vi "抓邊.vi"() -> ()   [LabVIEW 2015]
uses:
  <vilib>/vision/Measure.llb/Edge Options.ctl
  <vilib>/vision/Measure.llb/Edge Polarity.ctl
  <vilib>/vision/NI_Vision_Development_Module.lvlib
panel:
  out "degrees":sgl
  in  "單點":bool
  in  "Edge Options":T1={"Edge Polarity"=0, "Kernel Size"=3, "Width"=3, "Minimum Edge Strength"=10.0, "Interpolation Type"=enum."Bilinear Fixed", "Data Processing Method"=enum."Average"} {"Edge Polarity" items=["All Edges", "Rising Edges", "Falling Edges"]; "Minimum Edge Strength" format="%.2f"; "Width" step=2; "Kernel Size" step=2}
  in  "開圖":bool
  out "Gradient Information":dbl[][](graph)
  out "Line Segment":T3 {"Point 2"."Y" format="%.2f"; "Point 2"."X" format="%.2f"; "Point 1"."Y" format="%.2f"; "Point 1"."X" format="%.2f"}
  out "error out":errorcluster
  in  "Direction":T4(ring)
  in  "Process":u16(ring) items=["Get First Edge", "Get First + Last Edge", "Get All Edges", "Get Best Edge"]
  out "Line Profile":T5(graph)
  in  "Gap":i32=10
  out "Image":T6(plugin-control)
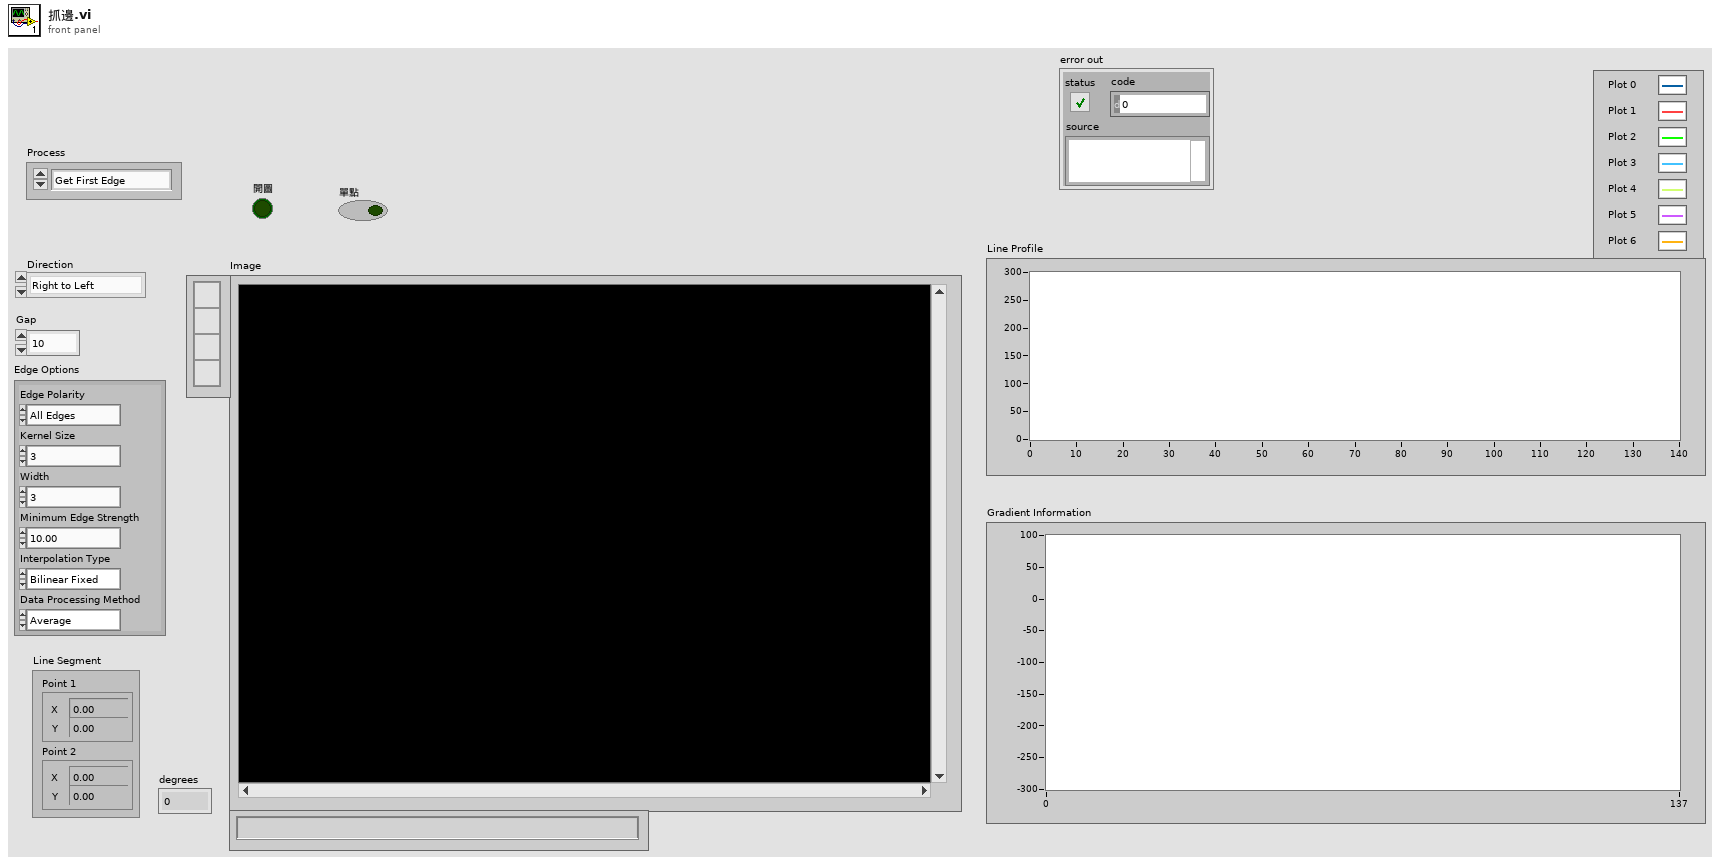
[diagram p1: front panel]
types:
  T1 = typedef "Edge Options.ctl" = cluster{"Edge Polarity":T2, "Kernel Size":u32, "Width":u32, "Minimum Edge Strength":sgl, "Interpolation Type":enum32{"Zero Order", "Bilinear", "Quadratic", "Cubic", "Bilinear Fixed"}, "Data Processing Method":enum32{"Average", "Median"}}
  T2 = typedef "Edge Polarity.ctl" = u32
  T3 = cluster{"Point 1":cluster{"X":sgl, "Y":sgl}, "Point 2":cluster{"X":sgl, "Y":sgl}}
  T4 = enum16{"Right to Left", "Left  to Right", "Up to Down", "Down to Up"}
  T5 = cluster{"x0":sgl, "dx":sgl, "Pixels Line":sgl[]}[]
  T6 = typedef "IMAQ Image.ctl" = refnum<image>
  T7 = typedef "Image Type" = u32
  T8 = cluster{"Global Rectangle":i32[], "Contours":cluster{"Contour Type":u32, "ROI Type":u32, "Points":i32[]}[]}
  T9 = typedef "IMAQ Line" = cluster{"Start X":i32, "Start Y":i32, "End X":i32, "End Y":i32}
  T10 = typedef "IMAQ Rectangle" = cluster{"Left":i32, "Top":i32, "Right":i32, "Bottom":i32, "Rotation":dbl}
  T11 = typedef "IMAQ Point" = cluster{"X":sgl, "Y":sgl}
  T12 = typedef "ROI Descriptor" = cluster{"Global Rectangle":i32[], "Contours":cluster{"ID":enum32{"External", "Internal"}, "Type":u32, "Coordinates":i32[]}[]}
  T13 = typedef "Edge New.ctl" = cluster{"Location (Pixel)":cluster{"X":sgl, "Y":sgl}, "Location (Real-World)":cluster{"X":sgl, "Y":sgl}, "Distance (Pixel)":dbl, "Distance (Real-World)":dbl, "Strength":dbl, "Noise":dbl, "Rising?":bool}
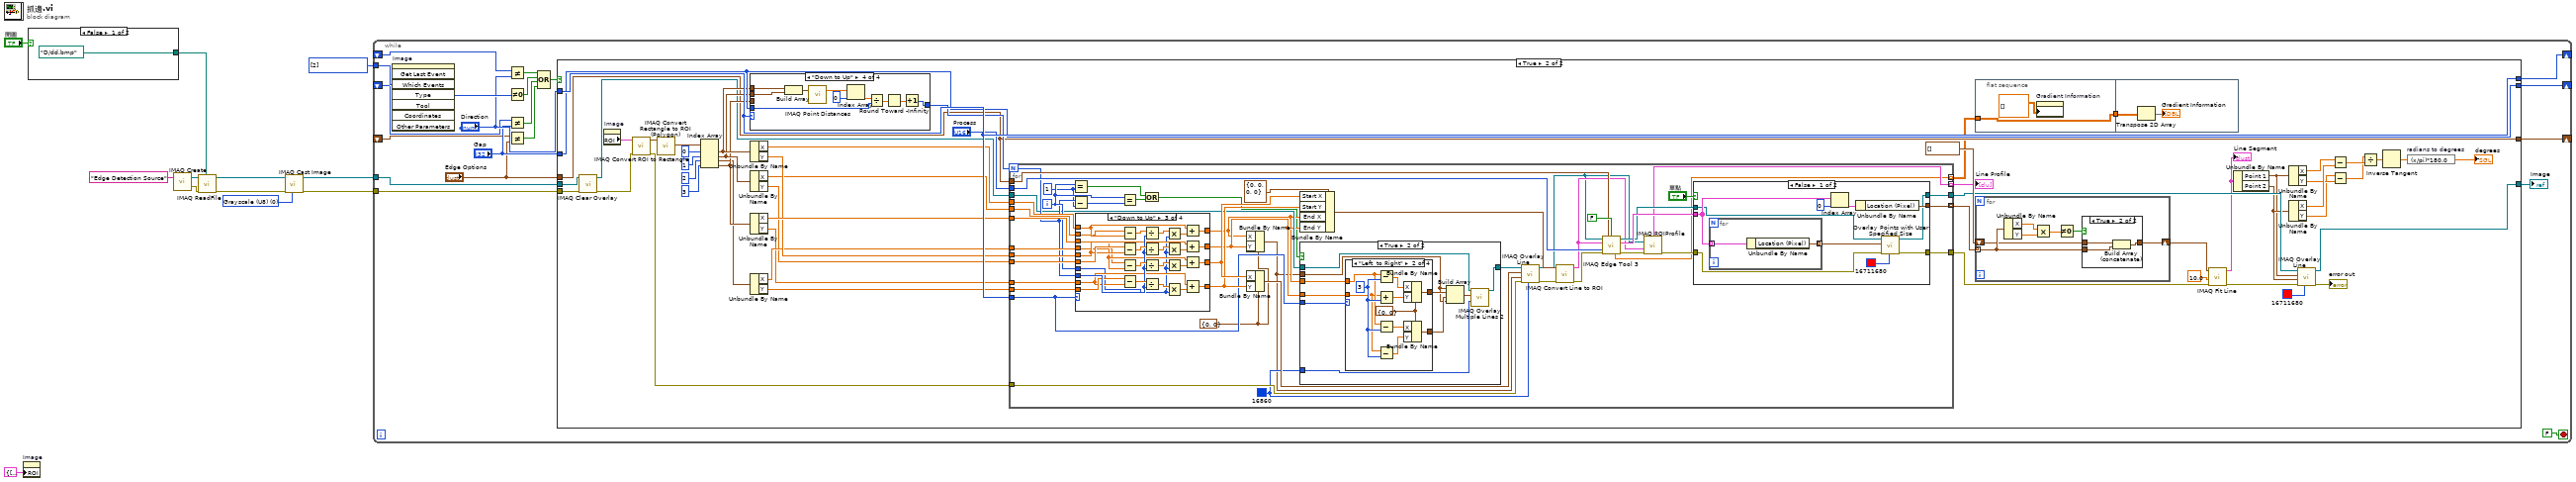
[diagram p0: block diagram]
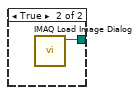
[diagram p2: hidden frame]
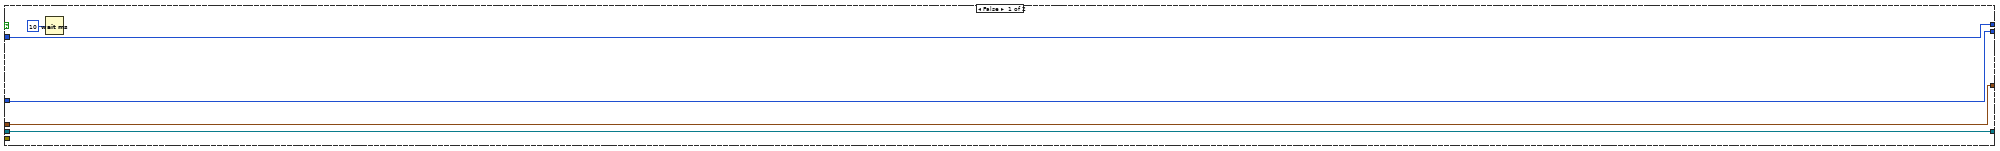
[diagram p3: hidden frame]
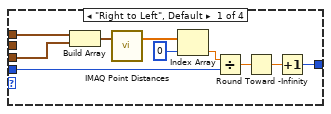
[diagram p4: hidden frame]
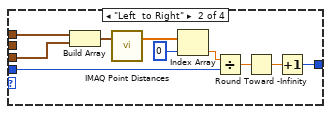
[diagram p5: hidden frame]
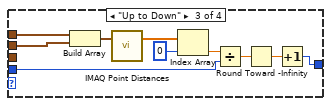
[diagram p6: hidden frame]
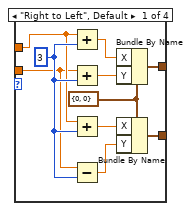
[diagram p9: hidden frame]
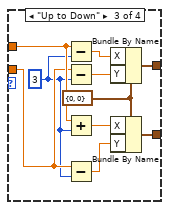
[diagram p10: hidden frame]
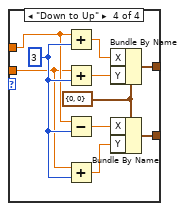
[diagram p11: hidden frame]
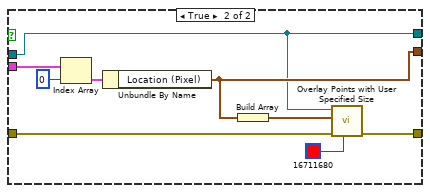
[diagram p12: hidden frame]
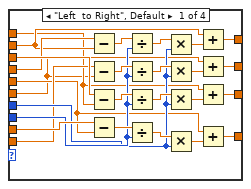
[diagram p13: hidden frame]
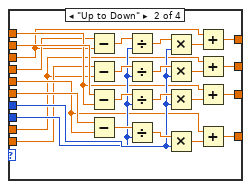
[diagram p14: hidden frame]
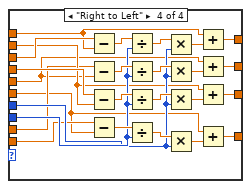
[diagram p15: hidden frame]
diagram:
  w6 = T7 0 items=["Grayscale (U8)", "Grayscale (I16)", "Grayscale (SGL)", "Complex (CSG)", "RGB (U32)", "HSL (U32)", "RGB (U64)", "Grayscale (U16)"] ("Image Type")
  w8 = i32[] [2] items=["No  event", "Click event", "Draw event", "Move event", "Size event", "Scroll event", "Activate event", "Close event", "Double click event"] ("Events list (all)")
  n1 = property on="Image" class="ImageControl"("ROI"=T8 {"Global Rectangle"=[450, 180, 600, 400], "Contours"=[{"Contour Type"=0, "ROI Type"=3, "Points"=[450, 180, 600, 400]}]}) -> ()  [unwired: 2 in, 2 out]
  n2 = case shown="False" "開圖" {
    tunnel: [path "D:/dd.bmp" ("File Path") w14] -> w3
    frame False {
    }
    frame True {
      n3 = call "IMAQ Load Image Dialog"() -> ("Path"=w14:path)  [unwired: 9 in, 2 out]
    }
  }
  n4 = call "IMAQ Create"("Image Name"="Edge Detection Source") -> ("New Image"=w11:T6, "error out"=w10:errorcluster)  [unwired: 4 in]
  n5 = call "IMAQ ReadFile"("File Path"=w3, "error in (no error)"=w10, "Image"=w11) -> ("error out"=w2:errorcluster, "Image Out"=w5:T6)  [unwired: 4 in, 3 out]
  n6 = call "IMAQ Cast Image"("Image Type"=w6, "error in (no error)"=w2, "Image Src"=w5) -> ("error out"=w1:errorcluster, "Image Dst Out"=w7:T6)  [unwired: 7 in]
  n7 = while {
    tunnel: w1 -> [w32]
    tunnel: w7 -> [w33]
    tunnel: w8 -> [w31]
    shift-right: [w29] -> _
    shift-left: _ -> [w28]
    shift-right: [w21] -> _
    shift-left: _ -> [w22]
    shift-right: [w16] -> _
    shift-left: _ -> [w17]
    stop <- FALSE stop-if-true
    n8 = invoke on="Image" class="ImageControl" method="Get Last Event"("Which Events"=w31) -> ("Type"=w30:i32)  [unwired: 7 in, 7 out]
    n9 = Not Equal?(x=w28, y="Direction") -> (x != y?=w27:bool)
    n10 = Not Equal To 0?(x=w30) -> (x != 0?=w26:bool)
    n11 = Not Equal?(x=w22, y="Gap") -> (x != y?=w20:bool)
    n12 = Not Equal?(x=w17, y="Edge Options") -> (x != y?=w15:bool)
    n13 = Compound Arithmetic op=OR(w27, w26, w20, w15) -> (w25:bool)
    n14 = case shown="True" w25 {
      tunnel: w33 -> [w36 w92]
      tunnel: w32 -> [_ w91]
      tunnel: "Direction" -> [w38 w82]
      tunnel: [w38 w82] -> w29
      tunnel: "Gap" -> [w37 w81]
      tunnel: [w37 w81] -> w21
      tunnel: [w36 w52] -> w19
      tunnel: "Edge Options" -> [w35 w61]
      tunnel: [w35 w61] -> w16
      frame False {
        n15 = Wait (ms)(milliseconds to wait=u32 10) -> ()  [unwired: 1 out]
      }
      frame True {
        n16 = call "IMAQ Clear Overlay"("error in (no error)"=w91, "Image"=w92) -> ("error out"=w90:errorcluster, "Image Out"=w64:T6)  [unwired: 8 in]
        n17 = property on="Image" class="ImageControl"() -> ("ROI"=w93:T8)  [unwired: 2 in, 2 out]
        n18 = call "IMAQ Convert ROI to Rectangle"("error in (no error)"=w90, "ROI Descriptor"=w93) -> ("error out"=w63:errorcluster, "Rectangle"=w85:T10)  [unwired: 7 in]
        n19 = call "IMAQ Convert Rectangle to ROI (Polygon)"("Rectangle"=w85) -> ("Rectangle Points"=w78:T11[])  [unwired: 7 in, 2 out]
        n20 = Index Array(array=w78, index #1=0 ("index"), index #2=1 ("index"), index #3=2 ("index"), index #4=3 ("index")) -> (element #1=w80:T11, element #2=w79:T11, element #3=w70:T11, element #4=w71:T11)
        n21 = case shown="\"Down to Up\"" w82 {
          tunnel: w81 -> [w101 w111 w121 w131]
          tunnel: [w100 w110 w120 w130] -> w77
          tunnel: w80 -> [w97 w107 w119 w127]
          tunnel: w71 -> [w96 w106 _ _]
          tunnel: w79 -> [_ _ w115 w126]
          frame "Right to Left", Default {
            n22 = Build Array(w97, w96) -> (w99:T11[])
            n23 = call "IMAQ Point Distances"("Points"=w99) -> ("Distances"=w98:sgl[])  [unwired: 4 in, 1 out]
            n24 = Index Array(array=w98, index=0) -> (element=w94:sgl)
            n25 = Divide(x=w94, y=w101) -> (x/y=w102:sgl)
            n26 = Round Toward -Infinity(1:w102) -> (0:w103:sgl)
            n27 = Increment(x=w103) -> (x+1=w100:i32)
          }
          frame "Left  to Right" {
            n28 = Build Array(w107, w106) -> (w109:T11[])
            n29 = call "IMAQ Point Distances"("Points"=w109) -> ("Distances"=w108:sgl[])  [unwired: 4 in, 1 out]
            n30 = Index Array(array=w108, index=0) -> (element=w104:sgl)
            n31 = Divide(x=w104, y=w111) -> (x/y=w112:sgl)
            n32 = Round Toward -Infinity(1:w112) -> (0:w113:sgl)
            n33 = Increment(x=w113) -> (x+1=w110:i32)
          }
          frame "Up to Down" {
            n34 = Build Array(w119, w115) -> (w118:T11[])
            n35 = call "IMAQ Point Distances"("Points"=w118) -> ("Distances"=w117:sgl[])  [unwired: 4 in, 1 out]
            n36 = Index Array(array=w117, index=0) -> (element=w116:sgl)
            n37 = Divide(x=w116, y=w121) -> (x/y=w122:sgl)
            n38 = Round Toward -Infinity(1:w122) -> (0:w123:sgl)
            n39 = Increment(x=w123) -> (x+1=w120:i32)
          }
          frame "Down to Up" {
            n40 = Build Array(w127, w126) -> (w129:T11[])
            n41 = call "IMAQ Point Distances"("Points"=w129) -> ("Distances"=w128:sgl[])  [unwired: 4 in, 1 out]
            n42 = Index Array(array=w128, index=0) -> (element=w125:sgl)
            n43 = Divide(x=w125, y=w131) -> (x/y=w132:sgl)
            n44 = Round Toward -Infinity(1:w132) -> (0:w133:sgl)
            n45 = Increment(x=w133) -> (x+1=w130:i32)
          }
        }
        n46 = Unbundle By Name(w80) -> ("X"=w75:sgl, "Y"=w74:sgl)
        n47 = Unbundle By Name(w79) -> ("X"=w68:sgl, "Y"=w66:sgl)
        n48 = Unbundle By Name(w71) -> ("X"=w76:sgl, "Y"=w65:sgl)
        n49 = Unbundle By Name(w70) -> ("X"=w69:sgl, "Y"=w67:sgl)
        n50 = for {
          N: w77 -> [w163]
          tunnel: w82 -> [w154]
          tunnel: w76 -> [w193]
          tunnel: w75 -> [w192]
          tunnel: w65 -> [w191]
          tunnel: w74 -> [w190]
          tunnel: w69 -> [w189]
          tunnel: w68 -> [w188]
          tunnel: w67 -> [w187]
          tunnel: w66 -> [w186]
          tunnel: [w175] -> w57
          tunnel: w64 -> [w158]
          tunnel: w63 -> [w184]
          tunnel: [w173] -> w56
          tunnel: "Process" -> [w176]
          tunnel: w61 -> [w172]
          tunnel: [w170] -> w60 mode=indexing
          tunnel: [w169] -> w59 mode=indexing
          tunnel: [w168] -> w58 mode=indexing
          i -> [w164]
          w162 = 1
          w156 = u32 16860 ("Color")
          w152 = cluster{"X":i32, "Y":i32} {"X"=0, "Y"=0} ("Start Point")
          n51 = Equal?(x=w164, y=w162) -> (x = y?=w160:bool)
          n52 = Subtract(x=w163, y=w162) -> (x-y=w161:i32)
          n53 = case shown="\"Down to Up\"" w154 {
            tunnel: [w277 w296 w322 w347] -> w183
            tunnel: [w272 w295 w321 w348] -> w151
            tunnel: [w275 w293 w319 w345] -> w182
            tunnel: [w271 w294 w320 w346] -> w153
            tunnel: w193 -> [w290 w301 w327 w357]
            tunnel: w192 -> [w268 w303 w326 w356]
            tunnel: w163 -> [w281 w305 w332 w358]
            tunnel: w164 -> [w280 w306 w323 w355]
            tunnel: w191 -> [w287 w297 w329 w352]
            tunnel: w190 -> [w270 w299 w328 w351]
            tunnel: w189 -> [w284 w302 w325 w354]
            tunnel: w188 -> [w269 w304 w324 w353]
            tunnel: w187 -> [w279 w298 w330 w350]
            tunnel: w186 -> [w267 w300 w331 w349]
            frame "Left  to Right", Default {
              n54 = Subtract(x=w284, y=w269) -> (x-y=w286:sgl)
              n55 = Subtract(x=w279, y=w267) -> (x-y=w282:sgl)
              n56 = Subtract(x=w290, y=w268) -> (x-y=w291:sgl)
              n57 = Subtract(x=w287, y=w270) -> (x-y=w289:sgl)
              n58 = Divide(x=w286, y=w281) -> (x/y=w285:sgl)
              n59 = Divide(x=w282, y=w281) -> (x/y=w283:sgl)
              n60 = Divide(x=w291, y=w281) -> (x/y=w292:sgl)
              n61 = Divide(x=w289, y=w281) -> (x/y=w288:sgl)
              n62 = Multiply(x=w285, y=w280) -> (x*y=w274:sgl)
              n63 = Multiply(x=w283, y=w280) -> (x*y=w273:sgl)
              n64 = Multiply(x=w292, y=w280) -> (x*y=w278:sgl)
              n65 = Multiply(x=w288, y=w280) -> (x*y=w276:sgl)
              n66 = Add(x=w269, y=w274) -> (x+y=w272:sgl)
              n67 = Add(x=w267, y=w273) -> (x+y=w271:sgl)
              n68 = Add(x=w268, y=w278) -> (x+y=w277:sgl)
              n69 = Add(x=w270, y=w276) -> (x+y=w275:sgl)
            }
            frame "Up to Down" {
              n70 = Subtract(x=w302, y=w301) -> (x-y=w314:sgl)
              n71 = Subtract(x=w298, y=w297) -> (x-y=w311:sgl)
              n72 = Subtract(x=w304, y=w303) -> (x-y=w317:sgl)
              n73 = Subtract(x=w300, y=w299) -> (x-y=w316:sgl)
              n74 = Divide(x=w314, y=w305) -> (x/y=w313:sgl)
              n75 = Divide(x=w311, y=w305) -> (x/y=w312:sgl)
              n76 = Divide(x=w317, y=w305) -> (x/y=w318:sgl)
              n77 = Divide(x=w316, y=w305) -> (x/y=w315:sgl)
              n78 = Multiply(x=w313, y=w306) -> (x*y=w308:sgl)
              n79 = Multiply(x=w312, y=w306) -> (x*y=w307:sgl)
              n80 = Multiply(x=w318, y=w306) -> (x*y=w310:sgl)
              n81 = Multiply(x=w315, y=w306) -> (x*y=w309:sgl)
              n82 = Add(x=w301, y=w308) -> (x+y=w295:sgl)
              n83 = Add(x=w297, y=w307) -> (x+y=w294:sgl)
              n84 = Add(x=w303, y=w310) -> (x+y=w296:sgl)
              n85 = Add(x=w299, y=w309) -> (x+y=w293:sgl)
            }
            frame "Down to Up" {
              n86 = Subtract(x=w324, y=w326) -> (x-y=w343:sgl)
              n87 = Subtract(x=w331, y=w328) -> (x-y=w342:sgl)
              n88 = Subtract(x=w325, y=w327) -> (x-y=w340:sgl)
              n89 = Subtract(x=w330, y=w329) -> (x-y=w337:sgl)
              n90 = Divide(x=w343, y=w332) -> (x/y=w344:sgl)
              n91 = Divide(x=w342, y=w332) -> (x/y=w341:sgl)
              n92 = Divide(x=w340, y=w332) -> (x/y=w339:sgl)
              n93 = Divide(x=w337, y=w332) -> (x/y=w338:sgl)
              n94 = Multiply(x=w344, y=w323) -> (x*y=w336:sgl)
              n95 = Multiply(x=w341, y=w323) -> (x*y=w335:sgl)
              n96 = Multiply(x=w339, y=w323) -> (x*y=w334:sgl)
              n97 = Multiply(x=w338, y=w323) -> (x*y=w333:sgl)
              n98 = Add(x=w326, y=w336) -> (x+y=w321:sgl)
              n99 = Add(x=w328, y=w335) -> (x+y=w320:sgl)
              n100 = Add(x=w327, y=w334) -> (x+y=w322:sgl)
              n101 = Add(x=w329, y=w333) -> (x+y=w319:sgl)
            }
            frame "Right to Left" {
              n102 = Subtract(x=w357, y=w356) -> (x-y=w369:sgl)
              n103 = Subtract(x=w352, y=w351) -> (x-y=w368:sgl)
              n104 = Subtract(x=w354, y=w353) -> (x-y=w366:sgl)
              n105 = Subtract(x=w350, y=w349) -> (x-y=w363:sgl)
              n106 = Divide(x=w369, y=w358) -> (x/y=w370:sgl)
              n107 = Divide(x=w368, y=w358) -> (x/y=w367:sgl)
              n108 = Divide(x=w366, y=w358) -> (x/y=w365:sgl)
              n109 = Divide(x=w363, y=w358) -> (x/y=w364:sgl)
              n110 = Multiply(x=w370, y=w355) -> (x*y=w362:sgl)
              n111 = Multiply(x=w367, y=w355) -> (x*y=w361:sgl)
              n112 = Multiply(x=w365, y=w355) -> (x*y=w360:sgl)
              n113 = Multiply(x=w364, y=w355) -> (x*y=w359:sgl)
              n114 = Add(x=w356, y=w362) -> (x+y=w348:sgl)
              n115 = Add(x=w351, y=w361) -> (x+y=w346:sgl)
              n116 = Add(x=w353, y=w360) -> (x+y=w347:sgl)
              n117 = Add(x=w349, y=w359) -> (x+y=w345:sgl)
            }
          }
          n118 = Equal?(x=w164, y=w161) -> (x = y?=w159:bool)
          n119 = Or(x=w160, y=w159) -> (x .or. y?=w149:bool)
          n120 = Bundle By Name(cluster=w152, "X"=w151, "Y"=w153) -> (w150:cluster{"X":i32, "Y":i32})
          n121 = Bundle By Name(cluster=w152, "X"=w183, "Y"=w182) -> (w185:cluster{"X":i32, "Y":i32})
          n122 = Bundle By Name(cluster=T9 {"Start X"=0, "Start Y"=0, "End X"=0, "End Y"=0} ("Line"), "Start X"=w183, "Start Y"=w182, "End X"=w151, "End Y"=w153) -> (w171:T9)
          n123 = case shown="True" w149 {
            tunnel: w158 -> [w195 w205]
            tunnel: [w195 w204] -> w157
            tunnel: w156 -> [_ w203]
            tunnel: w154 -> [_ w202]
            tunnel: w151 -> [_ w196]
            tunnel: w153 -> [_ w201]
            tunnel: w150 -> [_ w197]
            frame False {
            }
            frame True {
              n124 = case shown="\"Left  to Right\"" w202 {
                tunnel: w196 -> [w207 w219 w231 w239]
                tunnel: w201 -> [w206 w218 w230 w238]
                tunnel: [w209 w217 w228 w237] -> w200
                tunnel: [w208 w216 w227 w236] -> w199
                frame "Right to Left", Default {
                  w211 = cluster{"X":i32, "Y":i32} {"X"=0, "Y"=0} ("Start Point")
                  w210 = 3
                  n125 = Add(x=w207, y=w210) -> (x+y=w212:sgl)
                  n126 = Add(x=w206, y=w210) -> (x+y=w213:sgl)
                  n127 = Add(x=w207, y=w210) -> (x+y=w214:sgl)
                  n128 = Subtract(x=w206, y=w210) -> (x-y=w215:sgl)
                  n129 = Bundle By Name(cluster=w211, "X"=w212, "Y"=w213) -> (w209:cluster{"X":i32, "Y":i32})
                  n130 = Bundle By Name(cluster=w211, "X"=w214, "Y"=w215) -> (w208:cluster{"X":i32, "Y":i32})
                }
                frame "Left  to Right" {
                  w221 = cluster{"X":i32, "Y":i32} {"X"=0, "Y"=0} ("Start Point")
                  w220 = 3
                  n131 = Subtract(x=w219, y=w220) -> (x-y=w222:sgl)
                  n132 = Add(x=w218, y=w220) -> (x+y=w223:sgl)
                  n133 = Subtract(x=w219, y=w220) -> (x-y=w224:sgl)
                  n134 = Subtract(x=w218, y=w220) -> (x-y=w225:sgl)
                  n135 = Bundle By Name(cluster=w221, "X"=w222, "Y"=w223) -> (w217:cluster{"X":i32, "Y":i32})
                  n136 = Bundle By Name(cluster=w221, "X"=w224, "Y"=w225) -> (w216:cluster{"X":i32, "Y":i32})
                }
                frame "Up to Down" {
                  w229 = cluster{"X":i32, "Y":i32} {"X"=0, "Y"=0} ("Start Point")
                  w226 = 3
                  n137 = Subtract(x=w231, y=w226) -> (x-y=w232:sgl)
                  n138 = Subtract(x=w230, y=w226) -> (x-y=w233:sgl)
                  n139 = Add(x=w231, y=w226) -> (x+y=w234:sgl)
                  n140 = Subtract(x=w230, y=w226) -> (x-y=w235:sgl)
                  n141 = Bundle By Name(cluster=w229, "X"=w232, "Y"=w233) -> (w228:cluster{"X":i32, "Y":i32})
                  n142 = Bundle By Name(cluster=w229, "X"=w234, "Y"=w235) -> (w227:cluster{"X":i32, "Y":i32})
                }
                frame "Down to Up" {
                  w241 = cluster{"X":i32, "Y":i32} {"X"=0, "Y"=0} ("Start Point")
                  w240 = 3
                  n143 = Add(x=w239, y=w240) -> (x+y=w242:sgl)
                  n144 = Add(x=w238, y=w240) -> (x+y=w243:sgl)
                  n145 = Subtract(x=w239, y=w240) -> (x-y=w244:sgl)
                  n146 = Add(x=w238, y=w240) -> (x+y=w245:sgl)
                  n147 = Bundle By Name(cluster=w241, "X"=w242, "Y"=w243) -> (w237:cluster{"X":i32, "Y":i32})
                  n148 = Bundle By Name(cluster=w241, "X"=w244, "Y"=w245) -> (w236:cluster{"X":i32, "Y":i32})
                }
              }
              n149 = Build Array(w197, w200, w199, w197) -> (w198:cluster{"X":i32, "Y":i32}[])
              n150 = call "IMAQ Overlay Multiple Lines 2"("Image"=w205, "Line End Points"=w198, "Color"=w203) -> ("Image Out"=w204:T6)  [unwired: 11 in, 1 out]
            }
          }
          n151 = call "IMAQ Overlay Line"("Color"=w156, "error in (no error)"=w184, "End Point"=w150, "Start Point"=w185, "Image"=w157) -> ("error out"=w174:errorcluster, "Image Out"=w155:T6)  [unwired: 5 in]
          n152 = call "IMAQ Convert Line to ROI"("error in (no error)"=w174, "Line"=w171) -> ("error out"=w166:errorcluster, "ROI Descriptor"=w165:T12)  [unwired: 7 in]
          n153 = call "IMAQ Edge Tool 3"("Image"=w155, "Edge Options"=w172, "Optimized Mode"=FALSE, "ROI Descriptor"=w165, "Process"=w176, "error in (no error)"=w166) -> ("Image (duplicate)"=w178:T6, "Edge Information"=w181:T13[], "Gradient Values"=w169:dbl[], "error out"=w167:errorcluster)  [unwired: 5 in, 1 out]
          n154 = call "IMAQ ROIProfile"("error in (no error)"=w167, "ROI Descriptor"=w165, "Image"=w155) -> ("error out"=w180:errorcluster, "ROI Graph"=w170:cluster{"x0":sgl, "dx":sgl, "Pixels Line":sgl[]})  [unwired: 1 in, 3 out]
          n155 = case shown="False" "單點" {
            tunnel: [w247 w258] -> w175
            tunnel: w181 -> [w249 w265]
            tunnel: [w252 w262] -> w168
            tunnel: w180 -> [w251 w260]
            tunnel: [w250 w259] -> w173
            tunnel: w178 -> [w246 w258]
            frame False {
              n156 = for {
                tunnel: w249 -> [w257] mode=indexing
                tunnel: [w256] -> w248 mode=indexing
                n157 = Unbundle By Name(w257) -> ("Location (Pixel)"=w256:cluster{"X":sgl, "Y":sgl})
              }
              n158 = Index Array(array=w249, index=0) -> (element=w253:T13)
              n159 = Unbundle By Name(w253) -> ("Location (Pixel)"=w252:cluster{"X":sgl, "Y":sgl})
              n160 = call "Overlay Points with User Specified Size.vi"("Color"=u32 16711680, "error in"=w251, "Points"=w248, "Image In"=w246) -> ("error out"=w250:errorcluster, "Image Out"=w247:T6)  [unwired: 6 in]
            }
            frame True {
              n161 = Index Array(array=w265, index=0) -> (element=w263:T13)
              n162 = Unbundle By Name(w263) -> ("Location (Pixel)"=w262:cluster{"X":sgl, "Y":sgl})
              n163 = Build Array(w262) -> (w261:cluster{"X":sgl, "Y":sgl}[])
              n164 = call "Overlay Points with User Specified Size.vi"("Color"=u32 16711680, "error in"=w260, "Points"=w261, "Image In"=w258) -> ("error out"=w259:errorcluster)  [unwired: 6 in, 1 out]
            }
          }
        }
        "Line Profile" <- w60
        n165 = flat-sequence {
          tunnel: w59 -> [w134]
          tunnel: [w134] -> w86
          tunnel: w86 -> [w136]
          frame #0 {
            n166 = property on="Gradient Information" class="WFChart (strict)"("History Data"=dbl[][] []) -> ()  [unwired: 2 in, 2 out]
          }
          frame #1 {
            n167 = Transpose 2D Array(2D array=w136) -> (transposed array=→"Gradient Information":dbl[][])
          }
        }
        n168 = for {
          tunnel: w58 -> [w140] mode=indexing
          shift-right: [w139] -> w88
          shift-left: cluster{"X":sgl, "Y":sgl}[] [] -> [w138]
          n169 = Unbundle By Name(w140) -> ("X"=w144:sgl, "Y"=w143:sgl)
          n170 = Multiply(x=w144, y=w143) -> (x*y=w142:sgl)
          n171 = Not Equal To 0?(x=w142) -> (x != 0?=w141:bool)
          n172 = case shown="True" w141 {
            tunnel: w140 -> [_ w148]
            tunnel: [w145 w147] -> w139
            tunnel: w138 -> [w145 w146]
            frame False {
            }
            frame True {
              n173 = Build Array (concatenate)(w146, w148) -> (w147:cluster{"X":sgl, "Y":sgl}[])
            }
          }
        }
        n174 = call "IMAQ Fit Line"("error in (no error)"=w56, "Pixel Radius"=sgl 10.0, "Points"=w88) -> ("error out"=w54:errorcluster, "Line Segment"=w53:T3)  [unwired: 3 in, 4 out]
        "Line Segment" <- w53
        n175 = Unbundle By Name(w53) -> ("Point 1"=w40:cluster{"X":sgl, "Y":sgl}, "Point 2"=w41:cluster{"X":sgl, "Y":sgl})
        n176 = Unbundle By Name(w40) -> ("X"=w50:sgl, "Y"=w48:sgl)
        n177 = Unbundle By Name(w41) -> ("X"=w49:sgl, "Y"=w47:sgl)
        n178 = call "IMAQ Overlay Line"("Color"=u32 16711680, "error in (no error)"=w54, "End Point"=w41, "Start Point"=w40, "Image"=w57) -> ("error out"=→"error out":errorcluster, "Image Out"=w52:T6)  [unwired: 5 in]
        n179 = Subtract(x=w50, y=w49) -> (x-y=w46:sgl)
        n180 = Subtract(x=w47, y=w48) -> (x-y=w45:sgl)
        n181 = Divide(x=w45, y=w46) -> (x/y=w44:sgl)
        n182 = Inverse Tangent(1:w44) -> (0:w43:sgl)
        n183 = expression code="(x/pi)*180.0" "radians to degrees"(w43) -> (→"degrees":sgl)
      }
    }
    "Image" <- w19
  }
